vi "Periodic Tasks.vi"(8 "error in":errorcluster) -> ()   [LabVIEW 2011]
doc: "This VI runs in parallel to other tasks. It can contain as many user-defined periodic loops as you need. These can carry out PID or other sorts of timed response."
uses:
  <vilib>/Rock Robotics/SystemInterfaces/Utilities/FPGA_UtilitiesLED State.ctl
  <vilib>/Rock Robotics/SystemInterfaces/Utilities/FPGA_UtilitiesLED Source.ctl
  <vilib>/Rock Robotics/WPI/DriverStation/WPI_DriverStationRobotMode.ctl
  Robot Global Data.vi
panel:
  in  "Set RPM":dbl(slide) scale=0.0..4000.0
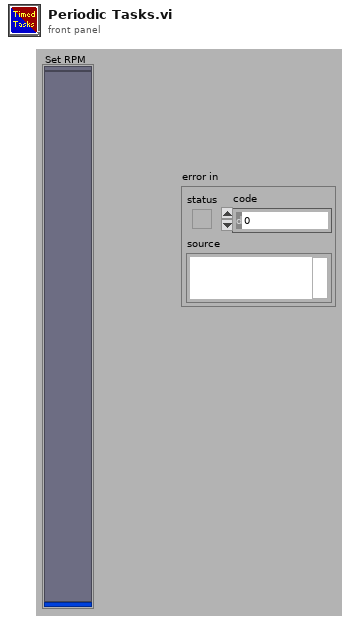
[diagram p1: front panel]
types:
  T1 = typedef "WPI_DriverStationRobotMode.ctl" = enum16{"Autonomous Disabled", "Autonomous Enabled", "Teleop Disabled", "Teleop Enabled", "Timeout", "Finish"}
  T2 = typedef "FPGA_UtilitiesLED State.ctl" = enum16{"Off", "On", "Toggle"}
  T3 = typedef "FPGA_UtilitiesLED Source.ctl" = enum16{"User LED", "FPGA LED"}
  T4 = cluster{cluster{"Ball Count Up":bool, "Ball Count Down":bool}, cluster{"Autonomous Delay":dbl, "Autonomous Mode":enum16{"Front Of Key", "Middle of Key (SEA)", "Back of Key", "Bridge", "Disable"}}}
  T5 = cluster{"Ball Count Up":bool, "Ball Count Down":bool}
  T6 = cluster{"Autonomous Delay":dbl, "Autonomous Mode":enum16{"Front Of Key", "Middle of Key (SEA)", "Back of Key", "Bridge", "Disable"}}
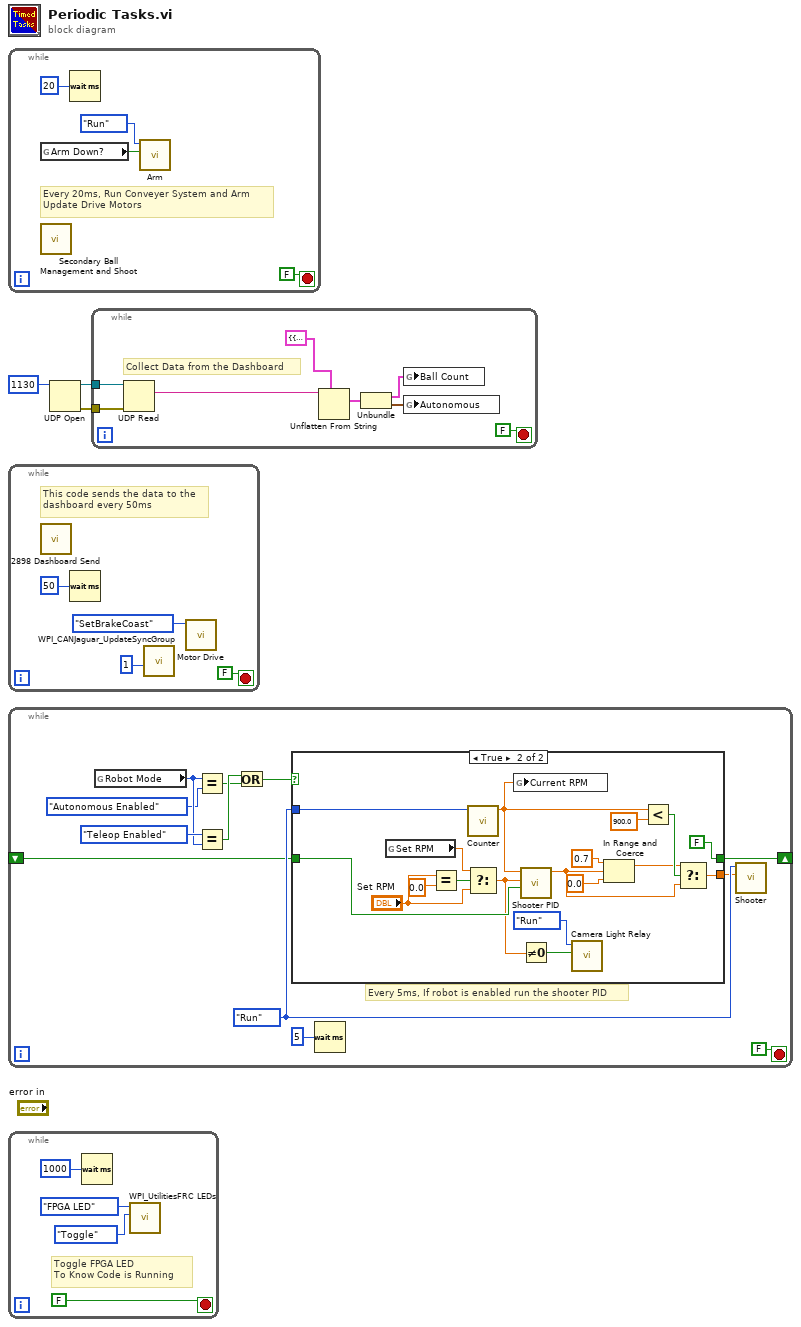
[diagram p0: block diagram]
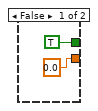
[diagram p2: hidden frame]
diagram:
  n1 = while {
    stop <- FALSE stop-if-true
    # "Every 20ms, Run Conveyer System and Arm\nUpdate Drive Motors"
    n2 = global read "Robot Global Data.vi" "Arm Down?"() -> (w5:bool)
    n3 = call "Secondary Ball Management and Shoot.vi"() -> ()  [unwired: 16 in]
    n4 = Wait (ms)(milliseconds to wait=u32 20) -> ()  [unwired: 1 out]
    n5 = call "Arm.vi"("Down?"=w5, "Enum"=enum16{"Init", "Run", "End"}."Run") -> ()  [unwired: 10 in]
  }
  n6 = while {
    stop <- FALSE stop-if-true
    # "This code sends the data to the\ndashboard every 50ms"
    n7 = call "2898 Dashboard Send.vi"() -> ()  [unwired: 12 in]
    n8 = Wait (ms)(milliseconds to wait=u32 50 ("millisecond multiple")) -> ()  [unwired: 1 out]
    n9 = call <vilib>:"WPI_CANJaguar_UpdateSyncGroup.vi"("Sync Group"=u8 1) -> ()  [unwired: 10 in, 1 out]
    n10 = call "Motor Drive.vi"("Enum"=enum16{"Init", "Run", "SetBrakeCoast", "End"}."SetBrakeCoast") -> ()  [unwired: 11 in]
  }
  n11 = while {
    shift-right: [w13] -> _
    shift-left: _ -> [w12]
    stop <- FALSE stop-if-true
    w22 = enum16{"Init", "Run", "End"}."Run" ("Enum")
    # "Every 5ms, If robot is enabled run the shooter PID"
    n12 = global read "Robot Global Data.vi" "Robot Mode"() -> (w20:T1)
    n13 = Equal?(x=w20, y=WPI_DriverStationRobotMode."Autonomous Enabled" ("Robot Mode")) -> (x = y?=w17:bool)
    n14 = Equal?(x=WPI_DriverStationRobotMode."Teleop Enabled" ("Robot Mode"), y=w20) -> (x = y?=w18:bool)
    n15 = Or(x=w18, y=w17) -> (x .or. y?=w16:bool)
    n16 = case shown="True" w16 {
      tunnel: w22 -> [_ w43]
      tunnel: [0.0 ("Motor") w34] -> w14
      tunnel: [TRUE FALSE] -> w13
      tunnel: w12 -> [_ w29]
      frame False {
      }
      frame True {
        n17 = global read "Robot Global Data.vi" "Set RPM"() -> (w39:dbl)
        n18 = Equal?(x="Set RPM", y=0.0) -> (x = y?=w41:bool)
        n19 = call "Counter.vi"("Enum"=w43) -> ("RPM"=w38:dbl)  [unwired: 10 in]
        n20 = Select(t=w39, s=w41, f="Set RPM") -> (s? t:f=w27:dbl)
        n21 = global write "Robot Global Data.vi" "Current RPM"(w38) -> ()
        n22 = call "Shooter PID.vi"("Current RPM"=w38, "Set RPM"=w27, "Reinitialize?"=w29) -> ("Motor"=w31:dbl)  [unwired: 7 in]
        n23 = Not Equal To 0?(x=w27) -> (x != 0?=w26:bool)
        n24 = call "Camera Light Relay.vi"("Camera Light"=w26, "Enum"=enum16{"Init", "Run", "End"}."Run") -> ()  [unwired: 10 in]
        n25 = In Range and Coerce(upper limit=0.7, x=w31, lower limit=0.0) -> (coerced(x)=w32:dbl)  [unwired: 1 out]
        n26 = Less?(x=w38, y=900.0) -> (x < y?=w33:bool)
        n27 = Select(t=w32, s=w33, f=w31) -> (s? t:f=w34:dbl)
      }
    }
    n28 = Wait (ms)(milliseconds to wait=u32 5) -> ()  [unwired: 1 out]
    n29 = call "Shooter.vi"("Enum"=w22, "Output"=w14) -> ()  [unwired: 9 in]
  }
  n30 = while {
    stop <- FALSE stop-if-true
    # "Toggle FPGA LED\nTo Know Code is Running"
    n31 = Wait (ms)(milliseconds to wait=u32 1000) -> ()  [unwired: 1 out]
    n32 = call <vilib>:"WPI_UtilitiesFRC LEDs.vi"("State"=FPGA_UtilitiesLED_State."Toggle", "LED Type"=FPGA_UtilitiesLED_Source."FPGA LED") -> ()  [unwired: 1 in, 9 out]
  }
  n33 = UDP Open(11:u16 1130 ("port")) -> (port=w2:refnum<k16>, 0:w1:errorcluster)  [unwired: 1 in, 4 out]
  n34 = while {
    tunnel: w2 -> [w54]
    tunnel: w1 -> [w53]
    stop <- FALSE stop-if-true
    # "Collect Data from the Dashboard"
    n35 = UDP Read(connection ID=w54, 8:w53) -> (data out=w52:string)  [unwired: 6 out]
    n36 = Unflatten From String(type=T4 {{"Ball Count Up"=FALSE, "Ball Count Down"=FALSE}, {"Autonomous Delay"=0.0, "Autonomous Mode"=enum."Middle of Key (SEA)"}} ("output cluster"), binary string=w52) -> (value=w51:T4)  [unwired: 2 in, 3 out]
    n37 = Unbundle(w51) -> (w48:T5, w49:T6)
    n38 = global write "Robot Global Data.vi" "Ball Count"(w48) -> ()
    n39 = global write "Robot Global Data.vi" "Autonomous"(w49) -> ()
  }
